vi "AD5781Deinit.vi"() -> (0 "timedOut":bool)   [LabVIEW 2014]
uses:
  Code/FPGA SPI_Globals.vi
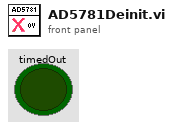
[diagram p1: front panel]
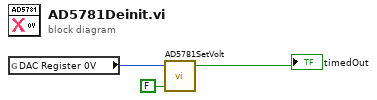
[diagram p0: block diagram]
diagram:
  n1 = global read "FPGA SPI_Globals.vi" "DAC Register 0V"() -> (w2:u32)
  n2 = call "AD5781SetVolt.vi"("Send"=FALSE, "SetVolt"=w2) -> ("timedOut"=→"timedOut":bool)  [unwired: 1 in, 2 out]
